vi "Verify with Multi Scrubber.vi"(8 "error in":errorcluster) -> (0 "error out":errorcluster)   [LabVIEW 2020, in "Caraya Extension Tests.lvclass"]
uses:
  Caraya Extension Tests.lvclass
  Caraya Extension Tests.lvclass/Caraya Extension Tests.ctl
  <vilib>/addons/_JKI Toolkits/Caraya/classes/Test/Test.lvclass
  4b862e9e-fcb2-487f-ab73-d9f83fbf4d2c.vi
  Source/Approval Tests/Regex Scrubber/Regex Scrubber.lvclass
  Source/Approval Tests/Options/Options.lvclass
  C:/Users/SAS/Desktop/ApprovalTests.LabVIEW/Source/Approval Tests/Regex Scrubber/Regex Scrubber.lvclass
  C:/Users/SAS/Desktop/ApprovalTests.LabVIEW/Source/Approval Tests/Scrubber/Scrubber.lvclass
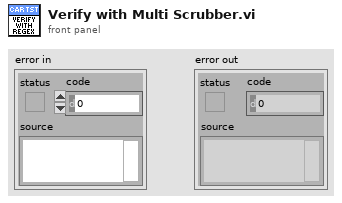
[diagram p1: front panel]
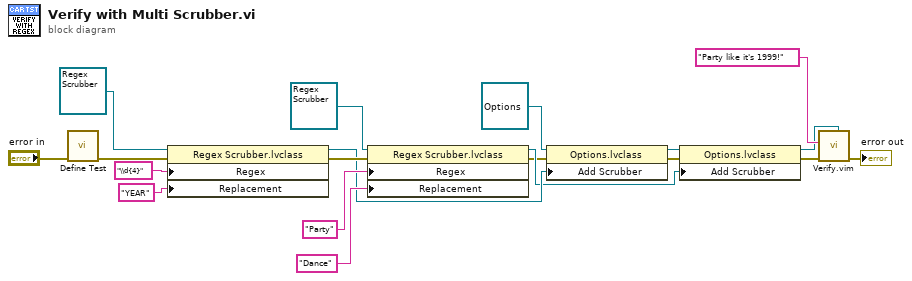
[diagram p0: block diagram]
diagram:
  n1 = call <vilib>:"Define Test.vi"("error in (no error)"="error in") -> ("error out"=w19:errorcluster)  [unwired: 9 in, 1 out]
  n2 = property class="Regex Scrubber.lvclass"(reference=refnum<class "Regex Scrubber.lvclass"> refnum ("Approval Tests.lvlib:Regex Scrubber.lvclass"), error in=w19, "Regex"="\\d{4}", "Replacement"="YEAR") -> (reference out=w7:refnum<class "Regex Scrubber.lvclass">, error out=w16:errorcluster)
  n3 = property class="Regex Scrubber.lvclass"(reference=refnum<class "Regex Scrubber.lvclass"> refnum ("Approval Tests.lvlib:Regex Scrubber.lvclass"), error in=w16, "Regex"="Party", "Replacement"="Dance") -> (reference out=w5:refnum<class "Regex Scrubber.lvclass">, error out=w4:errorcluster)
  n4 = property class="Options.lvclass"(reference=refnum<class "Options.lvclass"> refnum ("Approval Tests.lvlib:Options.lvclass"), error in=w4, "Add Scrubber"=w7) -> (reference out=w6:refnum<class "Options.lvclass">, error out=w3:errorcluster)
  n5 = property class="Options.lvclass"(reference=w6, error in=w3, "Add Scrubber"=w5) -> (reference out=w2:refnum<class "Options.lvclass">, error out=w1:errorcluster)
  n6 = call "Verify.vim"("Options"=w2, "error in"=w1, "Test Data"="Party like it's 1999!") -> ("error out"=→"error out":errorcluster)  [unwired: 8 in]
